vi "gyro -- sourcer async - V3 -- mfli.vi"(11 "sourcer event pair":T1) -> ()   [LabVIEW 2018]
uses:
  publisher action.ctl
  MFLI frontend action.ctl
  mfli reader event.ctl
  server talkto message type.ctl
  data source action.ctl
  PLL data source.ctl
  server talk-to-back pair.ctl
  server talkback message type.ctl
panel:
  in  "all":enum32{"all", "all 2"}(tab)
  out "read Voltage (V)":cdb=-1.5704114053890808e-07-1.022273978513787e-06i format="%#10_10f"
  in  "read OK":bool
  out "read Voltage X (V)":dbl=-1.5704114053890808e-07 format="%#11_11f"
  out "read Voltage Y (V)":dbl=-1.022273978513787e-06 format="%#11_11f"
  in  "delay-read (msec)":i64=20
  out "zi freq (Hz)":dbl=38764.725127578 format="%-#.3f"
  in  "amplitude (V)":dbl=0.001 format="%#_6p"
  in  "start  !":bool
  in  "stop  !":bool
  out "device selector":enum32{"MFLI"}(tab)
  in  "MFLI Address":string="DEV3523"
  in  "set amp!":bool
  in  "data rate (Sa/s)":dbl=100000.0 format="%#_6p"
  in  "set data rate!":bool
  out "Stopped?":bool=TRUE
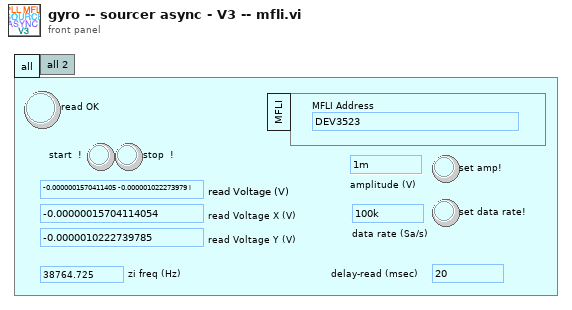
[diagram p1: front panel]
types:
  T1 = typedef "server talk-to-back pair.ctl" = cluster{"talkback event":refnum<user-event>, "talkto event":refnum<user-event>}
  T2 = typedef "MFLI frontend action.ctl" = enum16{"read", "writeread", "open", "close", "write"}
  T3 = typedef "server talkto message type.ctl" = cluster{"message":enum16{"stop", "start", "update pars", "update request", "new", "launch", "exit", "get", "reset", "pause", "unpause"}}
  T4 = typedef "mfli reader event.ctl" = enum16{"start", "stop", "exit", "set amplitude", "set datarate"}
  T5 = typedef "Zurich Instruments LabOne.lvlib/ziTypeHandle.ctl" = cluster{"handleValid":bool, "Conn":u64, "Path Prefix":string, "Handle":u64, "Connected":bool, "Clockbase(s)":dbl}
  T6 = typedef "publisher action.ctl" = enum16{"set", "get", "init", "check"}
  T7 = typedef "PLL data source.ctl" = enum16{"meta", "MFLI", "SRS865A", "arydh"}
  T8 = typedef "data source action.ctl" = enum16{"set", "get", "init", "set-and-get", "init source"}
  T9 = enum16{"stop", "start", "update pars", "update request", "new", "launch", "exit", "get", "reset", "pause", "unpause"}
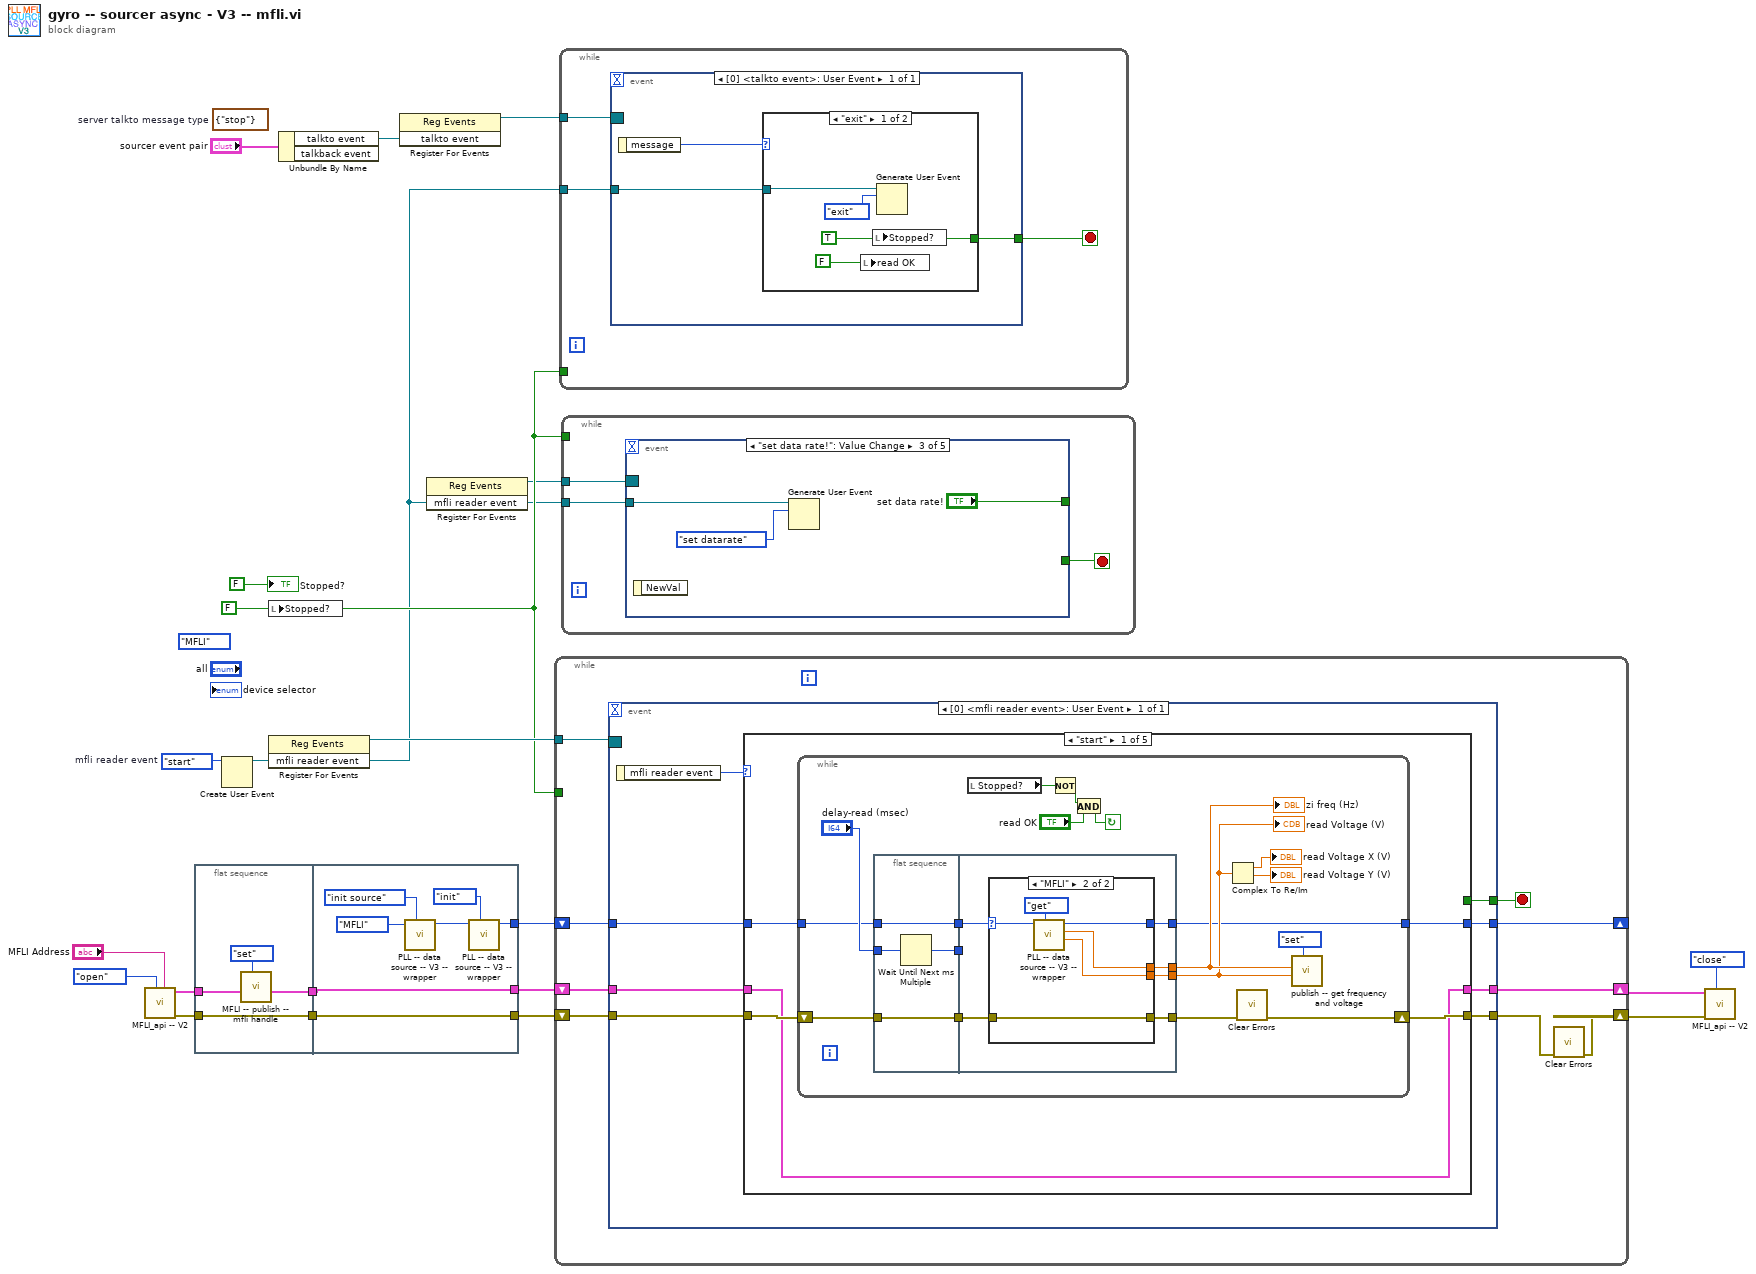
[diagram p0: block diagram]
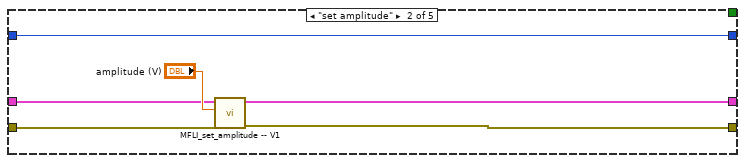
[diagram p4: hidden frame]
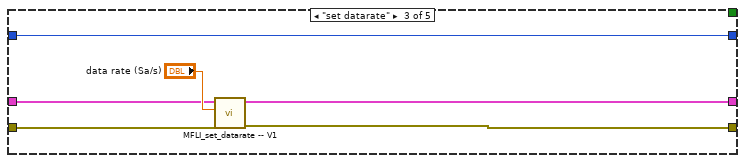
[diagram p5: hidden frame]
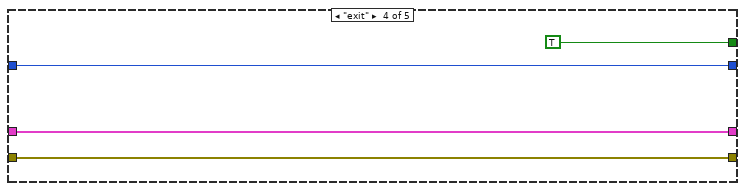
[diagram p6: hidden frame]
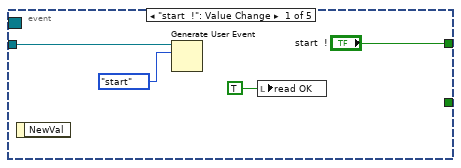
[diagram p8: hidden frame]
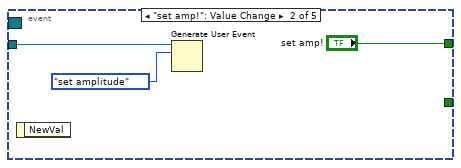
[diagram p9: hidden frame]
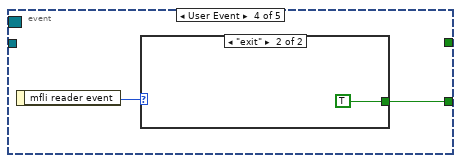
[diagram p10: hidden frame]
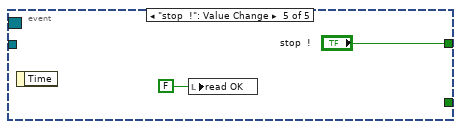
[diagram p12: hidden frame]
diagram:
  (unwired) enum32{"MFLI", "ARydh", "meta"}."MFLI" ("device selector")
  (unwired) T3 {"message"=enum."stop"}  # server talkto message type
  w13 = FALSE ("Stop")
  w20 = mfli_reader_event."start"  # mfli reader event
  n1 = call "MFLI_api -- V2.vi"("MFLI Address"="MFLI Address", "MFLI frontend action"=MFLI_frontend_action."open") -> ("Error Out"=w4:errorcluster, "Handle Out"=w6:T5)  [unwired: 6 in, 2 out]
  n2 = flat-sequence {
    tunnel: [w24] -> w9
    tunnel: w6 -> [w23]
    tunnel: [w22] -> w5
    tunnel: w4 -> [w22]
    tunnel: [w27] -> w18
    tunnel: [w29] -> w10
    tunnel: w9 -> [w26]
    tunnel: w5 -> [w27]
    tunnel: [w26] -> w2
    frame #0 {
      n3 = call "MFLI -- publish -- mfli handle.vi"("publisher action"=publisher_action."set", "Handle IN"=w23) -> ("Handle Out"=w24:T5)  [unwired: 9 in]
    }
    frame #1 {
      n4 = call "PLL -- data source -- V3 -- wrapper.vi"("data source action"=data_source_action."init source", "PLL data source"=PLL_data_source."MFLI") -> ("PLL data source OUT"=w32:T7)  [unwired: 7 in, 2 out]
      n5 = call "PLL -- data source -- V3 -- wrapper.vi"("data source action"=data_source_action."init", "PLL data source"=w32) -> ("PLL data source OUT"=w29:T7)  [unwired: 7 in, 2 out]
    }
  }
  n6 = Create User Event(user event datatype=w20) -> (user event=w11:refnum<user-event>)  [unwired: 1 in, 1 out]
  n7 = local write "Stopped?"(w13) -> ()
  n8 = register-events(w11) -> (reference out=w21:refnum<event-registration>)  [unwired: 2 in, 1 out]
  n9 = Unbundle By Name("sourcer event pair") -> ("talkto event"=w15:refnum<user-event>)  [unwired: 1 out]
  n10 = register-events(w15) -> (reference out=w17:refnum<event-registration>)  [unwired: 2 in, 1 out]
  n11 = register-events(w11) -> (reference out=w12:refnum<event-registration>)  [unwired: 2 in, 1 out]
  n12 = while {
    tunnel: w21 -> [w41]
    shift-right: [w33] -> w19
    shift-left: w18 -> [w40]
    tunnel: w13 -> [_]
    shift-right: [w37] -> _
    shift-left: w10 -> [w38]
    shift-right: [w35] -> w1
    shift-left: w2 -> [w36]
    stop <- w39 stop-if-true
    n13 = event shown="[0] <mfli reader event>: User Event" {
      selector: w41 -> [_]
      dyn-events: _ -> [_]
      timeout: _ -> [_]
      tunnel: w40 -> [w49]
      tunnel: [w48] -> w34
      tunnel: [w46] -> w39
      tunnel: w38 -> [w45]
      tunnel: [w44] -> w37
      tunnel: [w43] -> w35
      tunnel: w36 -> [w42]
      event User Event {
        n14 = event-data() -> ("mfli reader event"=w47:T4)  [unwired: 1 in]
        n15 = case shown="\"start\"" w47 {
          tunnel: w49 -> [w51 w96 w102 w106 w109]
          tunnel: [w54 w91 w97 w106 w109] -> w48
          tunnel: [_ _ _ TRUE _] -> w46
          tunnel: w45 -> [w53 w93 w99 w104 w108]
          tunnel: [w52 w93 w99 w104 w108] -> w44
          tunnel: [w50 w94 w100 w103 w107] -> w43
          tunnel: w42 -> [w50 w92 w98 w103 w107]
          frame "start" {
            n16 = while {
              shift-right: [w55] -> w54
              shift-left: w51 -> [w72]
              tunnel: w53 -> [w57]
              tunnel: [w59] -> w52
              stop <- w62 continue-if-true
              n17 = flat-sequence {
                tunnel: [w76] -> w71
                tunnel: "delay-read (msec)" -> [w75]
                tunnel: [w74] -> w70
                tunnel: w72 -> [w74]
                tunnel: [w73] -> w58
                tunnel: w57 -> [w73]
                tunnel: w71 -> [_]
                tunnel: [w80] -> w64
                tunnel: [w79] -> w65
                tunnel: w70 -> [w82]
                tunnel: [w81] -> w56
                tunnel: [w78] -> w59
                tunnel: w58 -> [w77]
                frame #0 {
                  n18 = Wait Until Next ms Multiple(millisecond multiple=w75) -> (millisecond timer value=w76:u32)
                }
                frame #1 {
                  n19 = case shown="\"MFLI\"" w77 {
                    selector: w77 -> [w83 w90]
                    tunnel: w82 -> [w84 w87]
                    tunnel: [w84 w87] -> w81
                    tunnel: [_ w86] -> w80
                    tunnel: [_ w85] -> w79
                    tunnel: [w83 w89] -> w78
                    frame "meta", Default {
                    }
                    frame "MFLI" {
                      n20 = call "PLL -- data source -- V3 -- wrapper.vi"("data source action"=data_source_action."get", "PLL data source"=w90) -> ("z out (V)"=w86:cdb, "Freq out (Hz)"=w85:dbl, "PLL data source OUT"=w89:T7)  [unwired: 7 in]
                    }
                  }
                }
              }
              n21 = local read "Stopped?"() -> (w60:bool)
              n22 = Not(x=w60) -> (.not. x?=w63:bool)
              n23 = And(x=w63, y="read OK") -> (x .and. y?=w62:bool)
              n24 = Complex To Re/Im(x + iy=w64) -> (x=→"read Voltage X (V)":dbl, y=→"read Voltage Y (V)":dbl)
              n25 = call <vilib>:"Clear Errors.vi"("error in (no error)"=w56) -> ("error out"=w55:errorcluster)  [unwired: 5 in, 1 out]
              n26 = call "publish -- get frequency and voltage.vi"("publisher action"=publisher_action."set", "Voltage IN (V)"=w64, "freq IN (Hz)"=w65) -> ()  [unwired: 6 in, 3 out]
              "read Voltage (V)" <- w64
              "zi freq (Hz)" <- w65
            }
          }
          frame "set amplitude" {
            n27 = call "MFLI_set_amplitude -- V1.vi"("Error In"=w96, "Amp in (V)"="amplitude (V)", "Handle In"=w92) -> ("Error Out"=w91:errorcluster, "Handle Out"=w94:T5)  [unwired: 5 in, 2 out]
          }
          frame "set datarate" {
            n28 = call "MFLI_set_datarate -- V1.vi"("Error In"=w102, "datarate (Sa/s) IN"="data rate (Sa/s)", "Handle In"=w98) -> ("Error Out"=w97:errorcluster, "Handle Out"=w100:T5)  [unwired: 5 in, 2 out]
          }
          frame "exit" {
          }
          frame "stop", Default {
          }
        }
      }
    }
    n29 = call <vilib>:"Clear Errors.vi"("error in (no error)"=w34) -> ("error out"=w33:errorcluster)  [unwired: 5 in, 1 out]
  }
  n30 = while {
    tunnel: w17 -> [w112]
    tunnel: w13 -> [_]
    tunnel: w11 -> [w110]
    stop <- w111 stop-if-true
    n31 = event shown="[0] <talkto event>: User Event" {
      selector: w112 -> [_]
      dyn-events: _ -> [_]
      timeout: _ -> [_]
      tunnel: [w114] -> w111
      tunnel: w110 -> [w113]
      event User Event {
        n32 = event-data() -> ("message"=w115:T9)  [unwired: 1 in]
        n33 = case shown="\"exit\"" w115 {
          tunnel: [w118 _] -> w114
          tunnel: w113 -> [w117 _]
          frame "exit" {
            w118 = TRUE ("Stoped?")
            n34 = local write "read OK"(FALSE ("read status")) -> ()
            n35 = local write "Stopped?"(w118) -> ()
            n36 = Generate User Event(user event=w117, event data cluster=mfli_reader_event."exit" ("event data")) -> ()  [unwired: 2 in, 2 out]
          }
          frame "get", Default {
          }
        }
      }
    }
  }
  n37 = while {
    tunnel: w11 -> [w122]
    tunnel: w13 -> [_]
    tunnel: w12 -> [w121]
    stop <- w120 stop-if-true
    n38 = event shown="[2] \"set data rate!\": Value Change" {
      selector: w121 -> [_ _ _ _ _]
      dyn-events: _ -> [_ _ _ _ _]
      timeout: _ -> [_ _ _ _ _]
      tunnel: ["start  !" "set amp!" "set data rate!" _ "stop  !"] -> _
      tunnel: w122 -> [w124 w129 w132 _ _]
      tunnel: [_ _ _ w133 _] -> w120
      event "start  !": Value Change {
        n39 = event-data() -> ()  [unwired: 1 in, 1 out]
        n40 = Generate User Event(user event=w124, event data cluster=mfli_reader_event."start" ("event data")) -> ()  [unwired: 2 in, 2 out]
        n41 = local write "read OK"(TRUE ("read status")) -> ()
      }
      event "set amp!": Value Change {
        n42 = event-data() -> ()  [unwired: 1 in, 1 out]
        n43 = Generate User Event(user event=w129, event data cluster=mfli_reader_event."set amplitude" ("event data")) -> ()  [unwired: 2 in, 2 out]
      }
      event "set data rate!": Value Change {
        n44 = event-data() -> ()  [unwired: 1 in, 1 out]
        n45 = Generate User Event(user event=w132, event data cluster=mfli_reader_event."set datarate" ("event data")) -> ()  [unwired: 2 in, 2 out]
      }
      event User Event {
        n46 = event-data() -> ("mfli reader event"=w134:T4)  [unwired: 1 in]
        n47 = case shown="\"exit\"" w134 {
          tunnel: [_ TRUE] -> w133
          frame "start", Default {
          }
          frame "exit" {
          }
        }
      }
      event "stop  !": Value Change {
        n48 = event-data() -> ()  [unwired: 1 in, 1 out]
        n49 = local write "read OK"(FALSE ("read status")) -> ()
      }
    }
  }
  n50 = call "MFLI_api -- V2.vi"("MFLI frontend action"=MFLI_frontend_action."close", "Error In"=w19, "Handle In"=w1) -> ()  [unwired: 5 in, 4 out]
  "Stopped?" <- FALSE ("Stoped?")
